vi "Move Step in Tree.vi"(9 "New Position":i32, 10 "Step Tag":string, 11 "TreeControl in":refnum<vi>) -> (3 "TreeControl out":refnum<vi>)   [LabVIEW 2020, in "Output Sequencer.lvlib" / "Settings UI.lvclass"]
uses:
  Settings UI.lvclass
  Types/Tree Index Enum.ctl
  Globals/Global Tree Data.vi
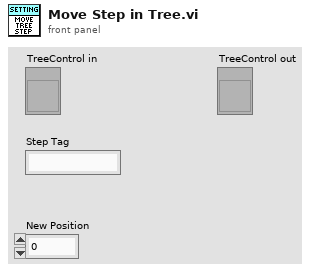
[diagram p1: front panel]
types:
  T1 = typedef "Output Sequencer.lvlib/Settings UI.lvclass/Tree Index Enum.ctl" = enum16{"General Settings", "Num Steps", "Num Analog", "Num Digital", "Show Confirmation", "Interp Priority", "Adv Timing", "Enable Conditions", "Seq Execution", "Reset Test Start", "Only When Test", "Delay After Test", "Start condition", "Re-triggering", "Stop condition", "Stop After Cycles", "Stop Values", "Default Values", "Default Analog", "Default Digital", "Steps", "Step #", "Description", "Precondition", "Duration", "Mode", "Delay Between Vals", "Analog Values", "Digital Values", "Postcondition", "On True", "On False"}
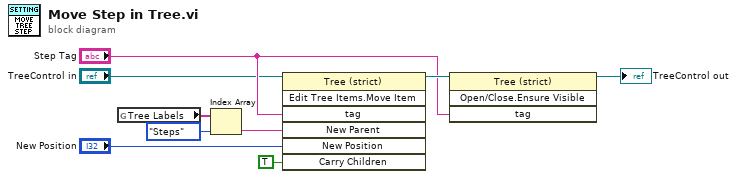
[diagram p0: block diagram]
diagram:
  n1 = global read "Global Tree Data.vi" "Tree Labels"() -> (w4:string[])
  n2 = Index Array(array=w4, index=Tree_Index_Enum."Steps" ("Tree Index Enum")) -> (element=w5:string)
  n3 = invoke class="Tree (strict)" method="Edit Tree Items.Move Item"(reference="TreeControl in", "tag"="Step Tag", "New Parent"=w5, "New Position"="New Position", "Carry Children"=TRUE ("Carry Children?")) -> (reference out=w7:refnum<vi>)  [unwired: 2 in, 6 out]
  n4 = invoke class="Tree (strict)" method="Open/Close.Ensure Visible"(reference=w7, "tag"="Step Tag") -> (reference out=→"TreeControl out":refnum<vi>)  [unwired: 2 in, 3 out]
